vi "str to accesstype.vi"(2 "String":string) -> (6 "access level":u16)   [LabVIEW 2013]
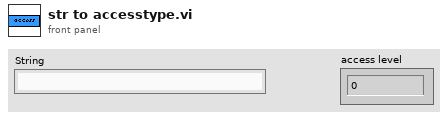
[diagram p1: front panel]
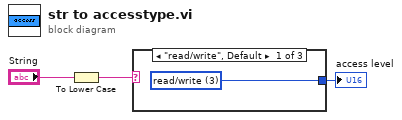
[diagram p0: block diagram]
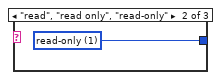
[diagram p2: hidden frame]
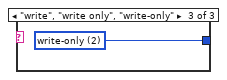
[diagram p3: hidden frame]
diagram:
  n1 = To Lower Case(string="String") -> (all lower case string=w2:string)
  n2 = case shown="\"read/write\", Default" w2 {
    tunnel: [w4 w5 w6] -> w1
    frame "read/write", Default {
      w4 = u16 3 items=["read-only"=1, "write-only"=2, "read/write"=3] ("access level")
    }
    frame "read", "read only", "read-only" {
      w5 = u16 1 items=["read-only"=1, "write-only"=2, "read/write"=3] ("access level")
    }
    frame "write", "write only", "write-only" {
      w6 = u16 2 items=["read-only"=1, "write-only"=2, "read/write"=3] ("access level")
    }
  }
  "access level" <- w1
